vi "McP Calibrate V0.80.vi"() -> ()   [LabVIEW 2021]
doc: "If you enter this program by mistake, click RETURN to quit.\n\nCALIBRATION STEPS:\n\n(0) Make sure you have calibration source (Ne lamp, Hg lamp, etc.) set up correctly.\n(1) Select a calibration line.\n(2) Click Calibrate.\n The spectrometer will move to the selected calibration line wavelength, take a CCD shot and fit the result.\n(3)Check the calibration result. You will be prompt whether to accept the result.\n (3a)Click \"Cancel\" to leave the system unaltered.\n (3b)If you click \"OK\", the counter position will be set to the calibrated value.\nThe spectrometer will return to the original internal (stepper) position afterward."
uses:
  Globals and TypeDefs/Global Varibal Control.vi
  Calibration/GlobalCalLampInfo.ctl
panel:
  in  "Return?":bool
  out "cursor position":dbl format="%.4f"
  in  "Points Between":i32=10 min=0 step=1
  out "Difference (cm-1)":dbl caption="(cm-1)" format="%.2e"
  out "Difference (meV)":dbl caption="(meV)" format="%.2e"
  out "Difference":dbl caption="(nm)" format="%.2e"
  out "Calibrated Wavelenth(nm)":dbl=1000.0 format="%.4f"
  out "peak plot (post-calibration)":cluster{"X-axis":dbl[], dbl[]}[](graph)
  out "Full plot":cluster{"X-axis":dbl[], "The Data":dbl[]}(graph)
  in  "Exposuretime (s)":dbl=0.5 format="%.2f"
  in  "CCD GPIB Address":u16=1
  in  "init CCD?":u16(ring) items=["Initialize the CCD camera", "The CCD has been initialized"]
  in  "init McP?":u16(ring) items=["Initialize the Spectrometer", "The spectrometer has been INITed"]
  out "Current WL":dbl=692.9467 caption="PreCalibrated Wavelength (nm)" format="%.4f"
  in  "Current Grating Density":enum16{"150", "300", "600", "1200", "1800"}(ring)=enum."1800"
  in  "Select WL":u16(ring)=6 caption="Select a Calibration Line" items=["808.2458  nm  ( Ne )", "794.3181  nm  ( Ne )", "743.8898  nm  ( Ne )", "724.5167  nm  ( Ne )", "717.3938  nm  ( Ne )", "703.2413  nm  ( Ne )", "692.9467  nm  ( Ne )", "671.7043  nm  ( Ne )", "667.8276  nm  ( Ne )", "659.8953  nm  ( Ne )", "653.2882  nm  ( Ne )", "650.6528  nm  ( Ne )", "640.2246  nm  ( Ne )", "638.2991  nm  ( Ne )", "633.4428  nm  ( Ne )", "632.8165  nm  ( Ne )", "579.2200  nm  ( Hg )", "577.1100  nm  ( Hg )", "546.2200  nm  ( Hg )", "435.9500  nm  ( Hg )", "407.8900  nm  ( Hg )", "404.7700  nm  ( Hg )", "366.4300  nm  ( Hg )", "365.5900  nm  ( Hg )", "365.1200  nm  ( Hg )", "Input Wavelength"]
  in  "StartCal":bool
  in  "Cal WL":dbl=692.9467 caption="Input Calibration Wavelength (nm)" format="%.4f"
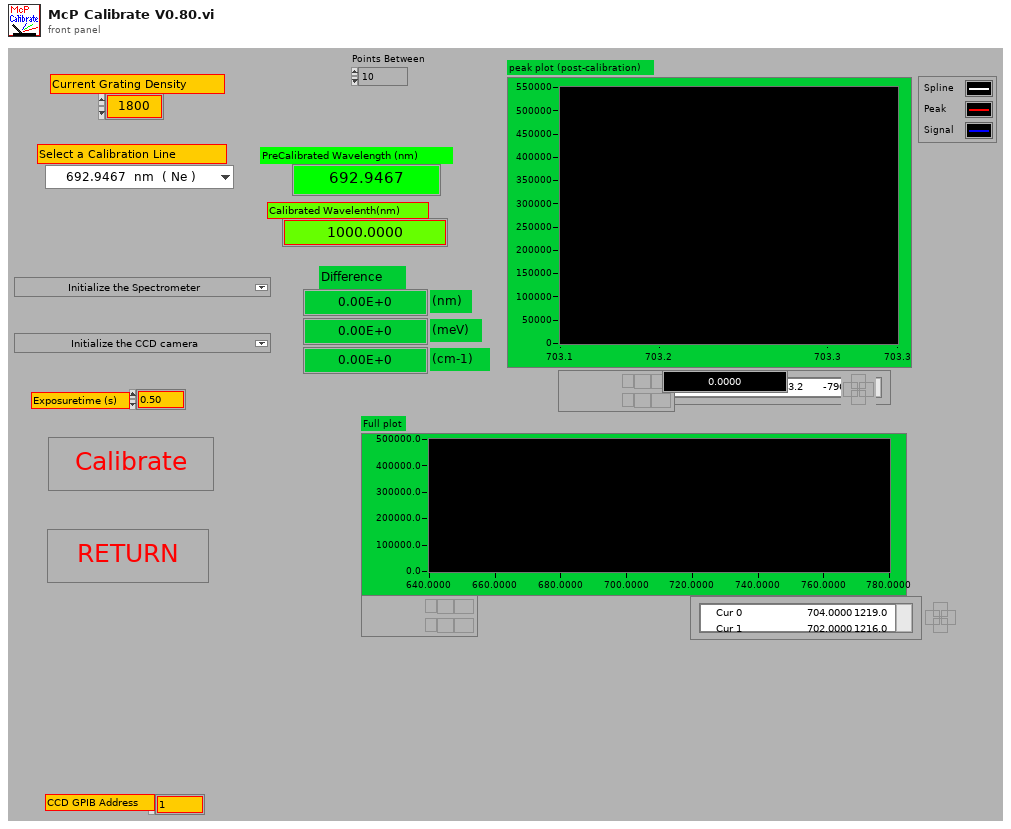
[diagram p1: front panel]
types:
  T1 = cluster{"Element":string, "Wavelength":dbl, "CalWidth":dbl}[]
  T2 = enum16{"Linear", "Polynomial", "Spline", "Rational"}
  T3 = cluster{"Element":string, "Wavelength":dbl, "CalWidth":dbl}
  T4 = typedef "McPhersonStatus.ctl" = enum16{"Ready", "+Slew", "-Slew", "Slew Done", "Begin Scan", "+Slew to Start", "-Slew to Start", "Scanning", "Scan Done", "Scan Pause", "Slew Pause"}
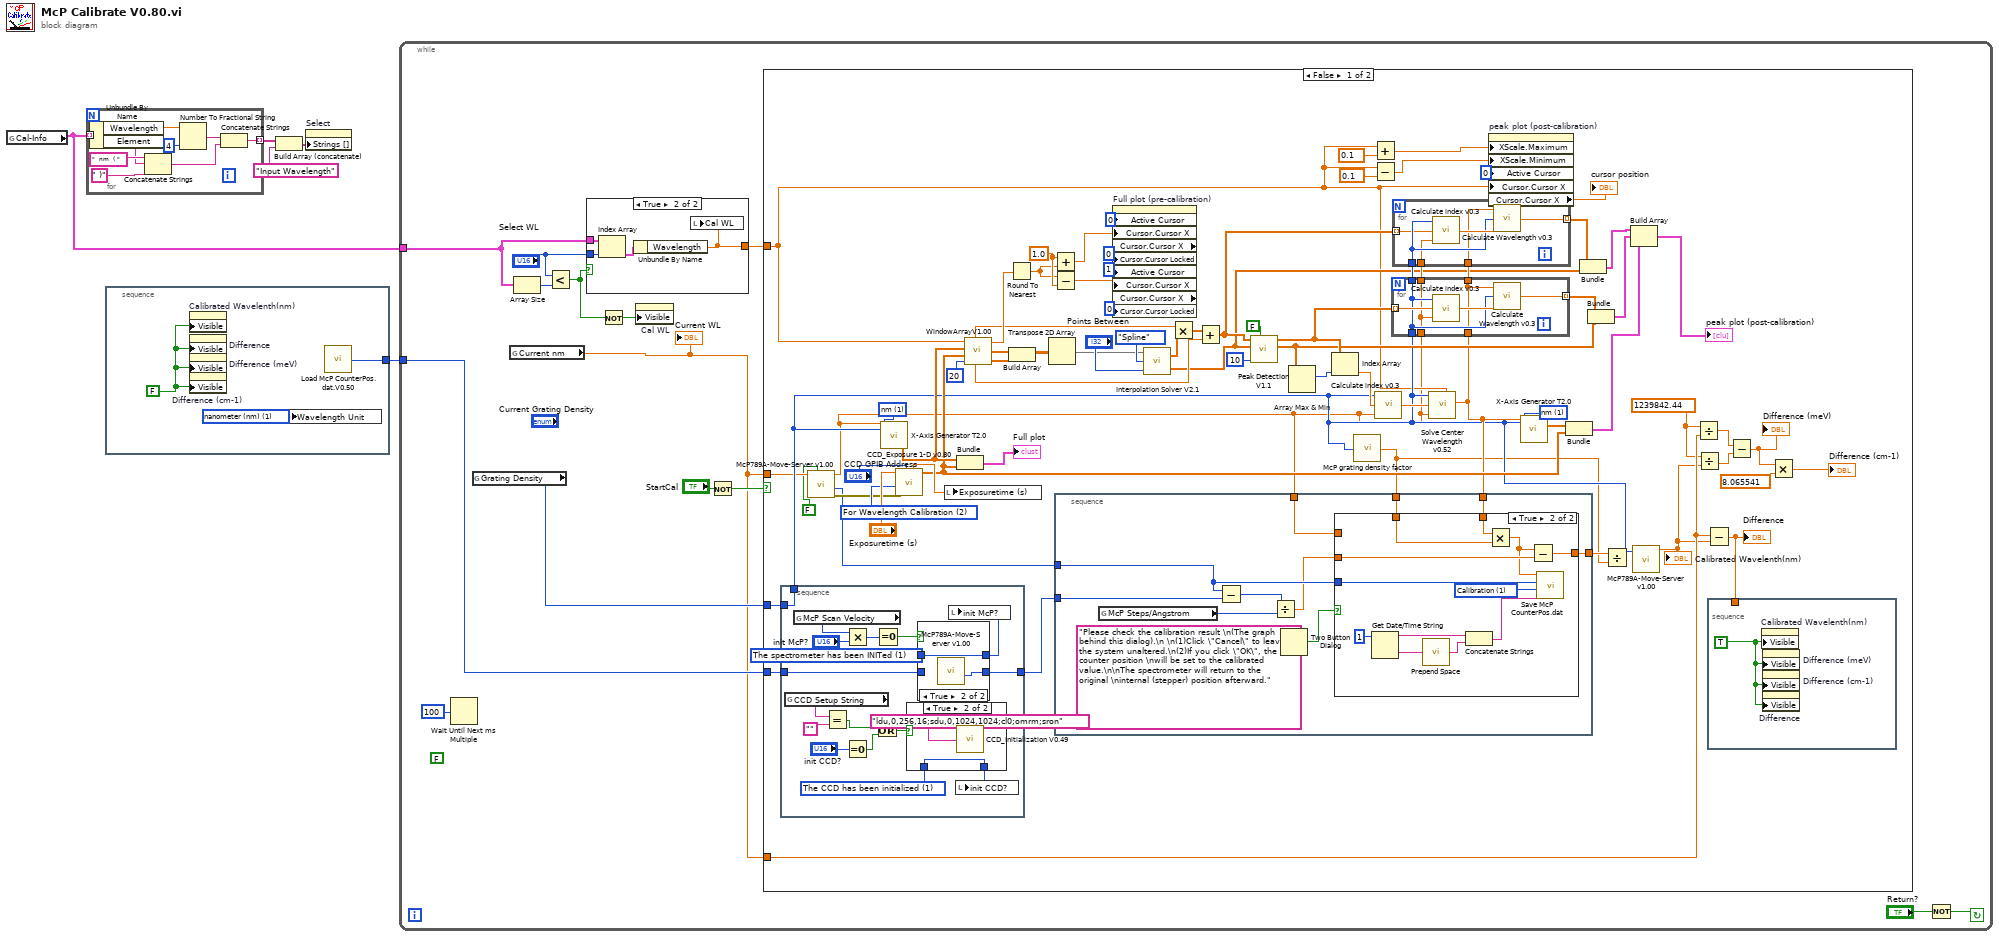
[diagram p0: block diagram]
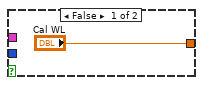
[diagram p2: hidden frame]
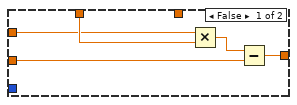
[diagram p3: hidden frame]
diagram:
  n1 = global read "GlobalCalLampInfo.ctl" "Cal-Info"() -> (w5:T1)
  n2 = for {
    tunnel: w5 -> [w14] mode=indexing
    tunnel: [w12] -> w4 mode=indexing
    n3 = Unbundle By Name(w14) -> ("Wavelength"=w11:dbl, "Element"=w8:string)
    n4 = Concatenate Strings("  nm  ( ", w8, " )") -> (w6:string)
    n5 = Number To Fractional String(number=w11, precision (6)=4) -> (F-format string=w10:string)  [unwired: 2 in]
    n6 = Concatenate Strings(w10, w6) -> (w12:string)
  }
  n7 = stacked-sequence {
    tunnel: [w17] -> w1
    frame #0 {
      w15 = u8 1 items=["Point #", "nanometer (nm)", "electron volt (eV)", "Milli eV (meV)", "Wavenumber (cm-1)"] ("Wavelength Unit")
      w16 = FALSE ("Visible")
      n8 = property on="Calibrated Wavelenth(nm)" class="DigNum (strict)"("Visible"=w16) -> ()  [unwired: 2 in, 2 out]
      n9 = property on="Difference" class="DigNum (strict)"("Visible"=w16) -> ()  [unwired: 2 in, 2 out]
      n10 = property on="Difference (meV)" class="DigNum (strict)"("Visible"=w16) -> ()  [unwired: 2 in, 2 out]
      n11 = property on="Difference (cm-1)" class="DigNum (strict)"("Visible"=w16) -> ()  [unwired: 2 in, 2 out]
      n12 = global write "Global Varibal Control.vi" "Wavelength Unit"(w15) -> ()
      n13 = call "Load McP CounterPos.dat.V0.50.vi"() -> ("Stepper Position"=w17:i32)  [unwired: 1 in, 2 out]
    }
  }
  n14 = Build Array (concatenate)(w4, "Input Wavelength") -> (w2:string[])
  n15 = property on="Select" class="Ring (strict)"("Strings []"=w2) -> ()  [unwired: 2 in, 2 out]
  n16 = while {
    tunnel: w1 -> [w29]
    tunnel: w5 -> [w31]
    stop <- w20 continue-if-true
    (unwired) FALSE
    n17 = Wait Until Next ms Multiple(millisecond multiple=u32 100) -> ()  [unwired: 1 out]
    n18 = global read "Global Varibal Control.vi" "Grating Density"() -> (w19:u8)
    n19 = global read "Global Varibal Control.vi" "Current nm"() -> (w18:dbl)
    "Current WL" <- w18
    n20 = Array Size(array=w31) -> (size(s)=w26:i32)
    n21 = Less?(x="Select WL", y=w26) -> (x < y?=w23:bool)
    n22 = case shown="True" w23 {
      tunnel: ["Cal WL" w34] -> w30
      tunnel: w31 -> [_ w35]
      tunnel: "Select WL" -> [_ w33]
      frame False {
      }
      frame True {
        n23 = Index Array(array=w35, index=w33) -> (element=w36:T3)
        n24 = Unbundle By Name(w36) -> ("Wavelength"=w34:dbl)
        n25 = local write "Cal WL"(w34) -> ()
      }
    }
    n26 = Not(x=w23) -> (.not. x?=w24:bool)
    n27 = property on="Cal WL" class="DigNum (strict)"("Visible"=w24) -> ()  [unwired: 2 in, 2 out]
    n28 = Not(x="StartCal") -> (.not. x?=w22:bool)
    n29 = case shown="False" w22 {
      tunnel: w30 -> [w41 _]
      tunnel: w18 -> [w45 _]
      tunnel: w29 -> [w52 _]
      tunnel: w19 -> [w51 _]
      tunnel: w18 -> [w40 _]
      frame False {
        w88 = 1 items=["Point #", "nm", "eV", "meV", "cm-1"] ("X-Axis Unit")
        w44 = 1239842.44
        w107 = 1.0
        w108 = 1 items=["Point #", "nm", "eV", "meV", "cm-1"] ("X-Axis Unit")
        w110 = u16 2 items=["No Over-Exposure Correction", "Over-Exposure Correction", "For Wavelength Calibration"] ("Mode")
        n30 = stacked-sequence {
          tunnel: w52 -> [w148]
          tunnel: [w147] -> w50
          tunnel: [w142] -> w43
          tunnel: w51 -> [w142]
          frame #0 {
            w143 = u16 1 items=["Initialize the CCD camera", "The CCD has been initialized"] ("init CCD?")
            w146 = u16 1 items=["Initialize the Spectrometer", "The spectrometer has been INITed"] ("init McP?")
            n31 = global read "Global Varibal Control.vi" "CCD Setup String"() -> (w153:string)
            n32 = global read "Global Varibal Control.vi" "McP Scan Velocity"() -> (w158:i32)
            n33 = Equal?(x=w153, y="") -> (x = y?=w151:bool)
            n34 = Multiply(x=w158, y="init McP?") -> (x*y=w156:i32)
            n35 = Equal To 0?(x="init CCD?") -> (x = 0?=w150:bool)
            n36 = Or(x=w151, y=w150) -> (x .or. y?=w149:bool)
            n37 = Equal To 0?(x=w156) -> (x = 0?=w155:bool)
            n38 = case shown="True" w149 {
              tunnel: [w159 w160] -> w144
              tunnel: w143 -> [w159 w160]
              frame False {
              }
              frame True {
                n39 = call "CCD_Initialization V0.49.vi"("Setup String"="ldu,0,256,16;sdu,0,1024,1024;cl0;omrm;sron") -> ()  [unwired: 4 in, 4 out]
              }
            }
            n40 = case shown="True" w155 {
              tunnel: w148 -> [w163 _]
              tunnel: [w163 w165] -> w147
              tunnel: [w162 w164] -> w145
              tunnel: w146 -> [w162 w164]
              frame False {
              }
              frame True {
                n41 = call "McP789A-Move-Server v1.00.vi"() -> ("ScanStatus"=w165:T4)  [unwired: 8 in, 2 out]
              }
            }
            n42 = local write "init McP?"(w145) -> ()
            n43 = local write "init CCD?"(w144) -> ()
          }
        }
        n44 = call "McP789A-Move-Server v1.00.vi"("Change Counter Position Manually"=FALSE ("Initializing MCP"), "GOTO"=w40) -> ("error out"=w109:errorcluster, "ScanStatus"=w94:T4, "CurrentPosition"=w39:dbl)  [unwired: 6 in]
        n45 = call "X-Axis Generator T2.0.vi"("Unit"=w43, "Grating Groove Density"=w108, "Central Wavelength"=w39) -> ("X-axis"=w99:dbl[])  [unwired: 3 out]
        n46 = call "CCD_Exposure 1-D v0.80.vi"("CCD GPIB Address"="CCD GPIB Address", "error in"=w109, "Mode"=w110, "Exposuretime (s)"="Exposuretime (s)") -> ("The Data"=w86:dbl[], "Exposuretime (s) out"=w93:dbl)  [unwired: 1 in, 5 out]
        n47 = local write "Exposuretime (s)"(w93) -> ()
        n48 = Bundle("X-axis"=w99, "The Data"=w86) -> (→"Full plot":cluster{"X-axis":dbl[], "The Data":dbl[]})  [unwired: 1 in]
        n49 = call "WindowArrayV1.00.vi"("Searching center"=w41, "X-axis"=w99, "The Data"=w86, "Window Width (point)"=20) -> ("scale"=w84:dbl, "starting point"=w83:dbl, "Closest peak position"=w98:dbl, "X-Axis Subset"=w70:dbl[], "Data Subset"=w69:dbl[])
        n50 = Round To Nearest(number=w98) -> (nearest integer value=w106:dbl)
        n51 = Build Array(w70, w69) -> (w72:dbl[][])
        n52 = Transpose 2D Array(2D array=w72) -> (transposed array=w71:dbl[][])
        n53 = Add(x=w107, y=w106) -> (x+y=w101:dbl)
        n54 = Subtract(x=w106, y=w107) -> (x-y=w100:dbl)
        n55 = property on="Full plot (pre-calibration)" class="XYGraph (strict)" props=["Active Cursor", "Cursor", "Cursor X", "Cursor", "Cursor X", "Cursor", "Cursor Locked", "Active Cursor", "Cursor", "Cursor X", "Cursor", "Cursor X", "Cursor", "Cursor Locked"]("Active Cursor"=u32 0, "Cursor.Cursor X"=w101, "Cursor.Cursor Locked"=u32 0 ("Cursor Locked"), "Active Cursor"=u32 1, "Cursor.Cursor X"=w100, "Cursor.Cursor Locked"=u32 0 ("Cursor Locked")) -> ()  [unwired: 2 in, 4 out]
        n56 = call "Interpolation Solver V2.1.vi"("Points Between"="Points Between", "Type of Interpolation"=T2."Spline", "Data"=w71) -> ("Interpolated Data"=w57:dbl[], "Interpolated X Axis"=w68:dbl[])
        n57 = Multiply(x=w84, y=w68) -> (x*y=w82:dbl[])
        n58 = Add(x=w82, y=w83) -> (x+y=w59:dbl[])
        n59 = call "Peak Detection V1.1.vi"("View Result?"=FALSE, "PD width"=10 ("Points Between"), "Input y data"=w57, "Input x data"=w59) -> ("Peak Amplitudes"=w56:dbl[], "Peak Locations"=w63:dbl[])  [unwired: 1 in, 5 out]
        n60 = Array Max & Min(array=w56) -> (max index (indices)=w81:i32)  [unwired: 3 out]
        n61 = Index Array(array=w63, index=w81) -> (element=w80:dbl)
        n62 = call "McP grating density factor.vi"("Grating Density"=w43) -> ("GratingFactor"=w42:dbl)
        n63 = Add(x=w41, y=0.1) -> (x+y=w76:dbl)
        n64 = Subtract(x=w41, y=0.1) -> (x-y=w75:dbl)
        n65 = call "Calculate index v0.3.vi"("Central Wavelength"=w39, "Current Wavelength"=w80, "Current Grating Density"=w43) -> ("index (out)"=w64:dbl)  [unwired: 2 in]
        n66 = call "Solve Center Wavelength v0.52.vi"("Standard Wavelength"=w41, "Current Central Wavelength"=w39, "pixel index"=w64, "Current Grating Density"=w43) -> ("Calibrated Central Wavelength"=w48:dbl)  [unwired: 4 in]
        n67 = stacked-sequence {
          tunnel: w94 -> [w123]
          tunnel: [w119] -> w46
          tunnel: w50 -> [w118]
          tunnel: w42 -> [w117]
          tunnel: w48 -> [w116]
          tunnel: w39 -> [w115]
          frame #0 {
            n68 = global read "Global Varibal Control.vi" "McP Steps/Angstrom"() -> (w121:i32)
            n69 = Subtract(x=w123, y=w118) -> (x-y=w122:i32)
            n70 = Divide(x=w122, y=w121) -> (x/y=w120:dbl)
            n71 = Two Button Dialog(message="Please check the calibration result \n(The graph behind this dialog).\n \n(1)Click \"Cancel\" to leave the system unaltered.\n(2)If you click \"OK\", the counter position \nwill be set to the calibrated value.\n\nThe spectrometer will return to the original \ninternal (stepper) position afterward.") -> (T button?=w114:bool)  [unwired: 2 in]
            n72 = case shown="True" w114 {
              tunnel: w123 -> [_ w140]
              tunnel: w120 -> [w126 w139]
              tunnel: [w127 w138] -> w119
              tunnel: w117 -> [w125 w131]
              tunnel: w116 -> [_ w130]
              tunnel: w115 -> [w124 _]
              frame False {
                n73 = Multiply(x=w124, y=w125) -> (x*y=w128:dbl)
                n74 = Subtract(x=w128, y=w126) -> (x-y=w127:dbl)
              }
              frame True {
                w137 = u16 1 items=["Moving", "Calibration", "Key in", "Initialization"] ("Set Method")
                n75 = Get Date/Time String(date format (0)=1) -> (date string=w133:string, time string=w135:string)  [unwired: 2 in]
                n76 = call "Prepend Space.vi"("Input String"=w135) -> ("Space + Input String"=w134:string)
                n77 = Concatenate Strings(w133, w134) -> (w132:string)
                n78 = Multiply(x=w130, y=w131) -> (x*y=w129:dbl)
                n79 = Subtract(x=w129, y=w139) -> (x-y=w138:dbl)
                n80 = call "Save McP CounterPos.dat.vi"("Last Calibration Date"=w132, "Set Method"=w137, "McP Stepper Position"=w140, "McP Counter Position"=w129) -> ()  [unwired: 2 in, 1 out]
              }
            }
          }
        }
        n81 = for {
          tunnel: w48 -> [w173]
          tunnel: w39 -> [w174]
          tunnel: w43 -> [w175]
          tunnel: w63 -> [w176] mode=indexing
          tunnel: [w175] -> w62
          tunnel: [w174] -> w60
          tunnel: [w173] -> w61
          tunnel: [w172] -> w55 mode=indexing
          n82 = call "Calculate index v0.3.vi"("Central Wavelength"=w174, "Current Wavelength"=w176, "Current Grating Density"=w175) -> ("index (out)"=w177:dbl)  [unwired: 2 in]
          n83 = call "Calculate Wavelength v0.3.vi"("pixel index"=w177, "Current Grating Density"=w175, "Central Wavelength"=w173) -> ("nm (out)"=w172:dbl)  [unwired: 2 in]
        }
        n84 = for {
          tunnel: w61 -> [w169]
          tunnel: w62 -> [w170]
          tunnel: w59 -> [w168] mode=indexing
          tunnel: w60 -> [w167]
          tunnel: [w166] -> w58 mode=indexing
          n85 = call "Calculate index v0.3.vi"("Central Wavelength"=w167, "Current Wavelength"=w168, "Current Grating Density"=w170) -> ("index (out)"=w171:dbl)  [unwired: 2 in]
          n86 = call "Calculate Wavelength v0.3.vi"("pixel index"=w171, "Current Grating Density"=w170, "Central Wavelength"=w169) -> ("nm (out)"=w166:dbl)  [unwired: 2 in]
        }
        n87 = property on="peak plot (post-calibration)" class="XYGraph (strict)"("XScale.Maximum"=w76, "XScale.Minimum"=w75, "Active Cursor"=u32 0, "Cursor.Cursor X"=w41) -> ("Cursor.Cursor X"=→"cursor position":dbl)  [unwired: 2 in, 2 out]
        n88 = call "X-Axis Generator T2.0.vi"("Unit"=w43, "Grating Groove Density"=w88, "Central Wavelength"=w48) -> ("X-axis"=w87:dbl[])  [unwired: 3 out]
        n89 = Bundle("X-axis"=w87, "The Data"=w86) -> (w79:cluster{"X-axis":dbl[], "The Data":dbl[]})  [unwired: 1 in]
        n90 = Bundle(w58, "Interpolated Data"=w57) -> (w67:cluster{dbl[], "Interpolated Data":dbl[]})  [unwired: 1 in]
        n91 = Bundle(w55, "Peak Amplitudes"=w56) -> (w66:cluster{dbl[], "Peak Amplitudes":dbl[]})  [unwired: 1 in]
        n92 = Divide(x=w46, y=w42) -> ()  [unwired: 1 out]
        n93 = Build Array(w67, w66, w79) -> (→"peak plot (post-calibration)":cluster{"X-axis":dbl[], "The Data":dbl[]}[])
        n94 = call "McP789A-Move-Server v1.00.vi"("GOTO"=w43) -> ("CurrentPosition"=w38:dbl)  [unwired: 7 in, 2 out]
        "Calibrated Wavelenth(nm)" <- w38
        n95 = Divide(x=w44, y=w45) -> (x/y=w92:dbl)
        n96 = Divide(x=w44, y=w38) -> (x/y=w91:dbl)
        n97 = Subtract(x=w45, y=w38) -> (x-y=w47:dbl)
        "Difference" <- w47
        n98 = stacked-sequence {
          tunnel: w47 -> [_]
          frame #0 {
            w141 = TRUE
            n99 = property on="Calibrated Wavelenth(nm)" class="DigNum (strict)"("Visible"=w141) -> ()  [unwired: 2 in, 2 out]
            n100 = property on="Difference (meV)" class="DigNum (strict)"("Visible"=w141) -> ()  [unwired: 2 in, 2 out]
            n101 = property on="Difference (cm-1)" class="DigNum (strict)"("Visible"=w141) -> ()  [unwired: 2 in, 2 out]
            n102 = property on="Difference" class="DigNum (strict)"("Visible"=w141) -> ()  [unwired: 2 in, 2 out]
          }
        }
        n103 = Subtract(x=w92, y=w91) -> (x-y=w90:dbl)
        "Difference (meV)" <- w90
        n104 = Multiply(x=w90, y=8.065541) -> (x*y=→"Difference (cm-1)":dbl)
      }
      frame True {
      }
    }
    n105 = Not(x="Return?") -> (.not. x?=w20:bool)
  }
